vi "Find Element.vi"(8 "error in (no error)":errorcluster, 10 "node Ref":refnum<data-value>, 11 "Priority Queue in":refnum<class "NI_Robotics_Priority Queue.lvclass">) -> (0 "error out":errorcluster, 2 "Numeric":i32, 3 "Priority Queue out":refnum<class "NI_Robotics_Priority Queue.lvclass">)   [LabVIEW 2017, in "NI_Robotics_Priority Queue.lvclass"]
uses:
  <vilib>/robotics/Navigation/shared/Priority Queue/NI_Robotics_Priority Queue.lvclass
  <vilib>/robotics/Navigation/shared/MapNode/AbstractMapNode/NI_Robotics_AbstractMapNode.lvclass
  <vilib>/robotics/Navigation/shared/Priority Queue/NI_Robotics_Priority Queue.lvclass/NI_Robotics_Priority Queue.ctl
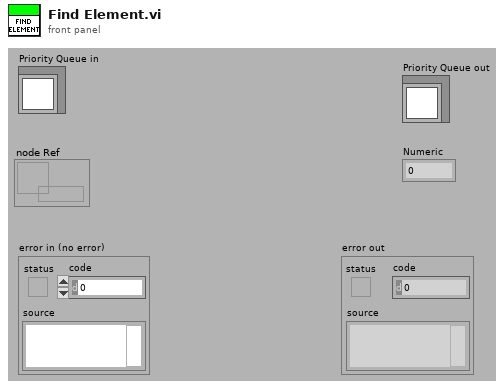
[diagram p1: front panel]
types:
  T1 = typedef "NI_Robotics_Priority Queue.lvclass/Open List Element.ctl" = cluster{"f":dbl, "g":dbl, "node Ref":refnum<data-value>}
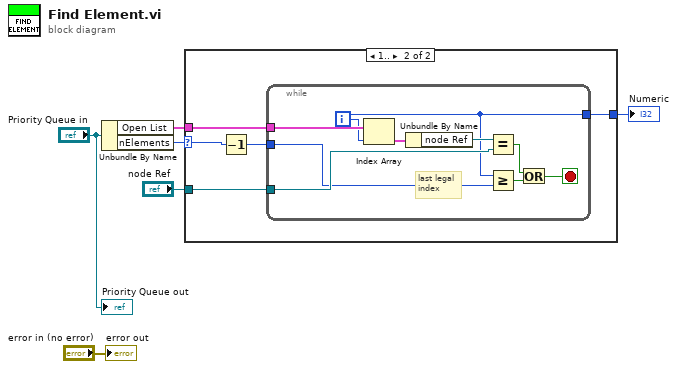
[diagram p0: block diagram]
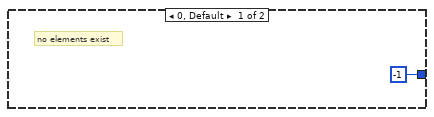
[diagram p2: hidden frame]
diagram:
  n1 = Unbundle By Name("Priority Queue in") -> ("Open List"=w6:T1[], "nElements"=w3:i32)
  n2 = case shown="1.." w3 {
    selector: w3 -> [_ w9]
    tunnel: w6 -> [_ w12]
    tunnel: "node Ref" -> [_ w11]
    tunnel: [-1 w10] -> w4
    frame 0, Default {
      # "no elements exist"
    }
    frame 1.. {
      n3 = Decrement(x=w9) -> (x-1=w8:i32)
      n4 = while {
        tunnel: w11 -> [w18]
        tunnel: [w14] -> w10
        tunnel: w12 -> [w21]
        tunnel: w8 -> [w13]
        i -> [w14]
        stop <- w17 stop-if-true
        # "last legal\nindex"
        n5 = Index Array(array=w21, index=w14) -> (element=w20:T1)
        n6 = Unbundle By Name(w20) -> ("node Ref"=w19:refnum<data-value>)
        n7 = Equal?(x=w19, y=w18) -> (x = y?=w16:bool)
        n8 = Greater Or Equal?(x=w14, y=w13) -> (x >= y?=w15:bool)
        n9 = Or(x=w16, y=w15) -> (x .or. y?=w17:bool)
      }
    }
  }
  "Numeric" <- w4
  "Priority Queue out" <- "Priority Queue in"
  "error out" <- "error in (no error)"
